vi "QCA - DUT Translate Tx Command.vi"(0 "TV Parameters(DataType)":T1 {"Tx_Chan" format="%.0x"; "Standard" items=["80211A/G/J/P OFDM", "80211B/G DSSS", "80211G DSSSOFDM", "80211N MIMOOFDM", "80211AC MIMOOFDM"]; "OFDM Data Rate (Mbps)" items=["6", "9", "12", "18", "24", "36", "48", "54"]; "80211n PLCP Frame Format" items=["Mixed Format", "Greenfield Format"]; "FEC Coding Type" items=["BCC", "LDPC"]; "DSSS Data Rate (Mbps)" items=["1", "2", "5.5 CCK", "5.5 PBCC", "11 CCK", "11 PBCC", "22", "33"]}, 5 "error in (no error)":errorcluster) -> (14 "Command Sent":string, 15 "FreqSet_f":i32, 16 "RateSet_r":i32[](array[numeric]), 17 "ChainSet_ch":i32, 18 "Standard_Index":i32, 19 "error out":errorcluster)   [LabVIEW 2011]
uses:
  TV/RW/Includes/WLAN - TV - RW - INC - TV_DataType_Cluster.ctl
  Controls/Transmit Config.ctl
  Controls/Data Rates.ctl
  Controls/Inter Frame Spacing modes.ctl
  Controls/Parameter.ctl
panel:
  in  "OFDM Data Rate (Mbps)":i32(ring) items=["6", "9", "12", "18", "24", "36", "48", "54"]
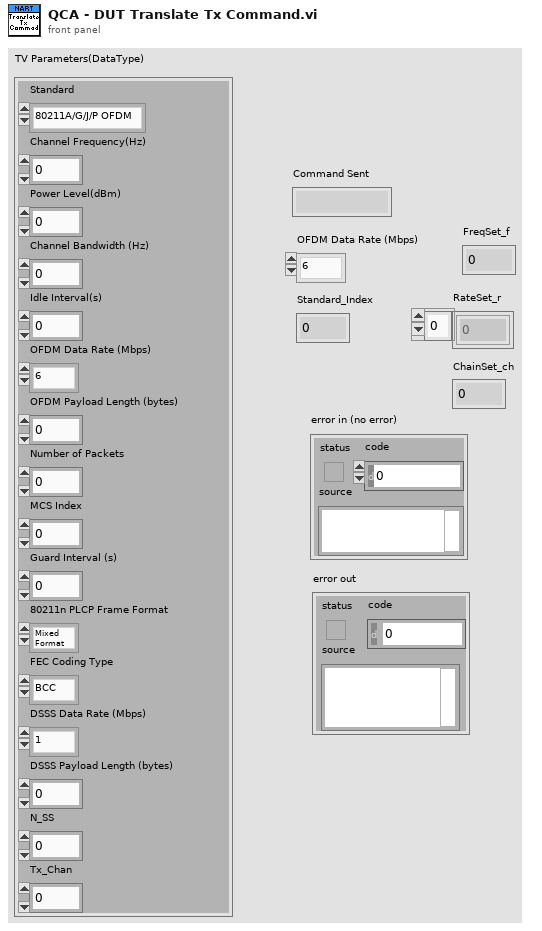
[diagram p1: front panel]
types:
  T1 = typedef "WLAN - TV - RW - INC - TV_DataType_Cluster.ctl" = cluster{"Standard":i32, "Channel Frequency(Hz)":dbl, "Power Level(dBm)":dbl, "Channel Bandwidth (Hz)":dbl, "Idle Interval(s)":dbl, "OFDM Data Rate (Mbps)":i32, "OFDM Payload Length (bytes)":i32, "Number of Packets":i32, "MCS Index":i32, "Guard Interval (s)":dbl, "80211n PLCP Frame Format":i32, "FEC Coding Type":i32, "DSSS Data Rate (Mbps)":i32, "DSSS Payload Length (bytes)":i32, "N_SS":i32, "Tx_Chan":u32}
  T2 = typedef "Data Rates.ctl" = string
  T3 = typedef "Transmit Config.ctl" = cluster{"Packet Length":u32, "Packet Count":i32, "Data Rate":T2, "Frequency, MHz":u32, "Continuous Frames":bool, "TX Power, dB":dbl}
  T4 = enum16{"none", "combined", "isolated", "iterate-combined ", "iterate-isolated"}
  T5 = typedef "Parameter.ctl" = cluster{"Name":string, "Type":enum16{"decimal", "string", "float", "hex"}}
  T6 = typedef "Inter Frame Spacing modes.ctl" = i16
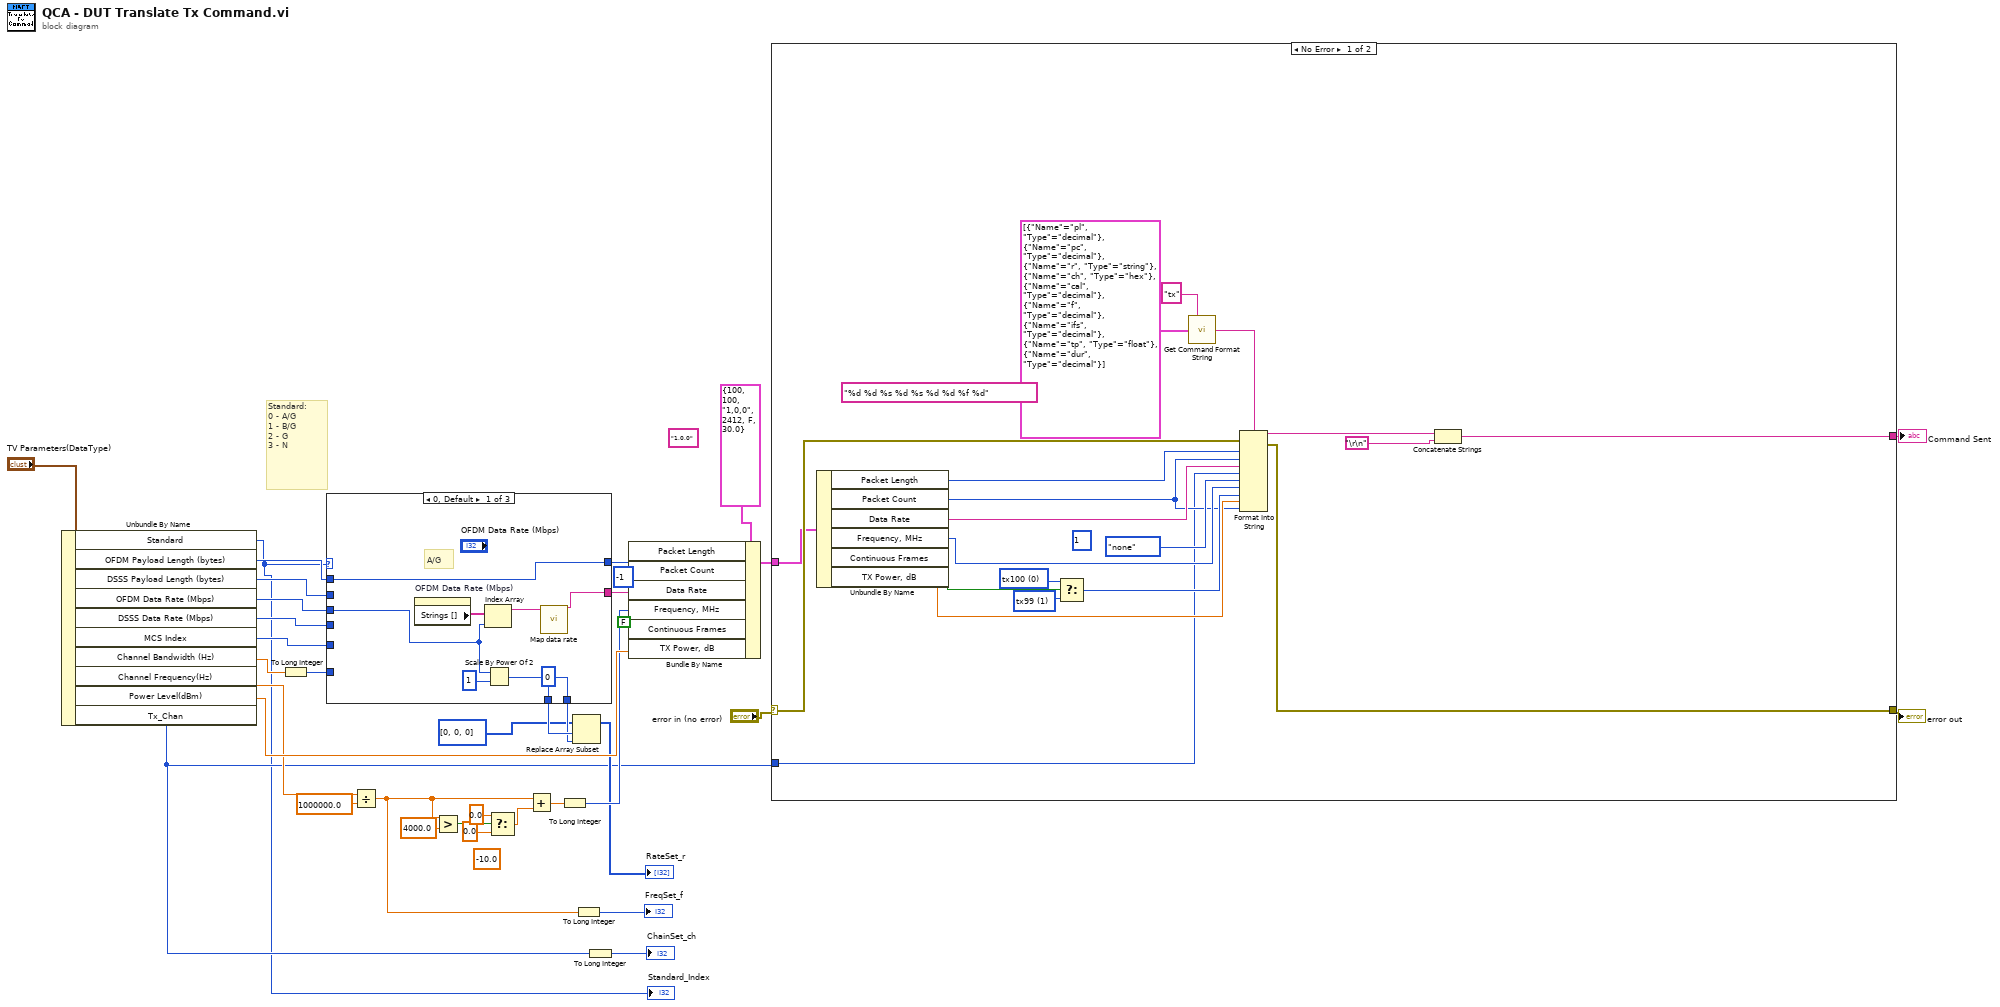
[diagram p0: block diagram]
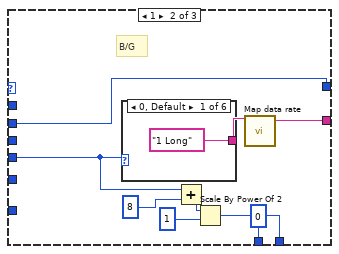
[diagram p2: hidden frame]
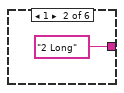
[diagram p3: hidden frame]
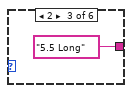
[diagram p4: hidden frame]
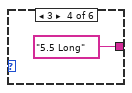
[diagram p5: hidden frame]
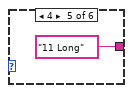
[diagram p6: hidden frame]
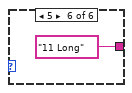
[diagram p7: hidden frame]
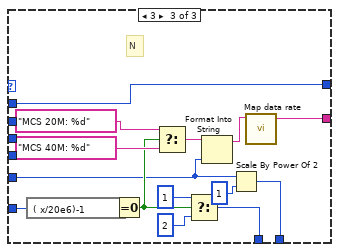
[diagram p8: hidden frame]
diagram:
  (unwired) -10.0 ("t")
  (unwired) T2 "1,0,0" ("Data Rate")
  # "Standard:\n0 - A/G\n1 - B/G\n2 - G\n3 - N"
  n1 = Unbundle By Name("TV Parameters(DataType)") -> ("Standard"=w1:i32, "OFDM Payload Length (bytes)"=w27:i32, "DSSS Payload Length (bytes)"=w26:i32, "OFDM Data Rate (Mbps)"=w25:i32, "DSSS Data Rate (Mbps)"=w23:i32, "MCS Index"=w22:i32, "Channel Bandwidth (Hz)"=w19:dbl, "Channel Frequency(Hz)"=w6:dbl, "Power Level(dBm)"=w24:dbl, "Tx_Chan"=w4:u32)
  "Standard_Index" <- w1
  n2 = To Long Integer(number=w19) -> (32bit integer=w18:i32)
  n3 = case shown="0, Default" w1 {
    tunnel: [w44 w53 w74] -> w28
    tunnel: w27 -> [w44 _ w74]
    tunnel: w26 -> [_ w53 _]
    tunnel: w25 -> [w40 _ _]
    tunnel: w23 -> [_ w46 _]
    tunnel: w22 -> [_ _ w61]
    tunnel: [w43 w52 w73] -> w21
    tunnel: w18 -> [_ _ w67]
    tunnel: [0 0 w63] -> w10
    tunnel: [w37 w48 w60] -> w9
    frame 0, Default {
      # "A/G"
      n4 = property on="OFDM Data Rate (Mbps)" class="Ring (strict)"() -> ("Strings []"=w42:string[])  [unwired: 2 in, 2 out]
      n5 = Index Array(array=w42, index=w40) -> (element=w41:string)
      n6 = Scale By Power Of 2(n=w40, x=1) -> (x*2^n=w37:i32)
      n7 = call "Map data rate.vi"("Data Rate In"=w41) -> ("Data Rate Out"=w43:string)  [unwired: 10 in]
    }
    frame 1 {
      # "B/G"
      n8 = case shown="0, Default" w46 {
        tunnel: ["1 Long" ("Data Rate In") "2 Long" ("Data Rate In") "5.5 Long" ("Data Rate In") "5.5 Long" ("Data Rate In") "11 Long" ("Data Rate In") "11 Long" ("Data Rate In")] -> w51
        frame 0, Default {
        }
        frame 1 {
        }
        frame 2 {
        }
        frame 3 {
        }
        frame 4 {
        }
        frame 5 {
        }
      }
      n9 = Add(x=w46, y=8) -> (x+y=w45:i32)
      n10 = Scale By Power Of 2(n=w45, x=1) -> (x*2^n=w48:i32)
      n11 = call "Map data rate.vi"("Data Rate In"=w51) -> ("Data Rate Out"=w52:string)  [unwired: 10 in]
    }
    frame 3 {
      # "N"
      n12 = expression code="( x/20e6)-1"(w67) -> (w71:i32)
      n13 = Equal To 0?(x=w71) -> (x = 0?=w66:bool)
      n14 = Select(t="MCS 20M: %d" ("format string"), s=w66, f="MCS 40M: %d" ("format string")) -> (s? t:f=w72:string)
      n15 = Select(t=1, s=w66, f=2) -> (s? t:f=w63:i32)
      n16 = Format Into String(format string=w72, w61) -> (resulting string=w68:string)  [unwired: 2 in, 1 out]
      n17 = Scale By Power Of 2(n=w61, x=1) -> (x*2^n=w60:i32)
      n18 = call "Map data rate.vi"("Data Rate In"=w68) -> ("Data Rate Out"=w73:string)  [unwired: 10 in]
    }
  }
  n19 = Divide(x=w6, y=1000000.0 ("x")) -> (x/y=w2:dbl)
  n20 = Greater?(x=w2, y=4000.0) -> (0:w16:bool)
  n21 = Select(t=0.0, s=w16, f=0.0) -> (s? t:f=w12:dbl)
  n22 = Add(x=w2, y=w12) -> (x+y=w13:dbl)
  n23 = To Long Integer(number=w13) -> (32bit integer=w11:i32)
  n24 = Replace Array Subset(array=i32[] [0, 0, 0], new element=w9, index=w10) -> (→"RateSet_r":i32[])
  n25 = To Long Integer(number=w2) -> (32bit integer=→"FreqSet_f":i32)
  n26 = To Long Integer(number=w4) -> (32bit integer=→"ChainSet_ch":i32)
  n27 = Bundle By Name(cluster=T3 {"Packet Length"=100, "Packet Count"=100, "Data Rate"="1,0,0", "Frequency, MHz"=2412, "Continuous Frames"=FALSE, "TX Power, dB"=30.0} ("Transmit Config"), "Packet Length"=w28, "Packet Count"=-1, "Data Rate"=w21, "Frequency, MHz"=w11, "Continuous Frames"=FALSE, "TX Power, dB"=w24) -> (w32:T3)
  n28 = case shown="No Error" "error in (no error)" {
    selector: "error in (no error)" -> [w94 w95]
    tunnel: [w76 w95] -> w35
    tunnel: [w87 _] -> w34
    tunnel: w32 -> [w77 _]
    tunnel: w4 -> [w75 _]
    frame No Error {
      (unwired) "%d %d %s %d %s %d %d %f %d" ("format string")
      w82 = T6 1 items=["Regular"=-1, "tx100"=0, "tx99"=1] ("ART2 Data.Transmit Config.Inter Frame Spacing")
      w83 = T6 0 items=["Regular"=-1, "tx100"=0, "tx99"=1] ("ART2 Data.Transmit Config.Inter Frame Spacing")
      (unwired) u32 1 ("Chains")
      n29 = Unbundle By Name(w77) -> ("Packet Length"=w93:u32, "Packet Count"=w79:i32, "Data Rate"=w85:T2, "Frequency, MHz"=w90:u32, "Continuous Frames"=w81:bool, "TX Power, dB"=w88:dbl)
      n30 = Select(t=w83, s=w81, f=w82) -> (s? t:f=w80:T6)
      n31 = call "Get Command Format String.vi"("Command"="tx", "Parameters"=T5[] [{"Name"="pl", "Type"=enum."decimal"}, {"Name"="pc", "Type"=enum."decimal"}, {"Name"="r", "Type"=enum."string"}, {"Name"="ch", "Type"=enum."hex"}, {"Name"="cal", "Type"=enum."decimal"}, {"Name"="f", "Type"=enum."decimal"}, {"Name"="ifs", "Type"=enum."decimal"}, {"Name"="tp", "Type"=enum."float"}, {"Name"="dur", "Type"=enum."decimal"}]) -> ("Command Format String"=w89:string)  [unwired: 13 in]
      n32 = Format Into String(format string=w89, error in=w94, w93, w79, w85, w75, T4."none" ("input 5"), w90, w80, w88, w79) -> (resulting string=w78:string, error out=w76:errorcluster)  [unwired: 1 in]
      n33 = Concatenate Strings(w78, "\r\n") -> (w87:string)
    }
    frame Error {
    }
  }
  "error out" <- w35
  "Command Sent" <- w34
